vi "Get Completed Log Files.vi"(8 "error in (no error)":errorcluster, 10 "Session Name in":string, 11 "Data Logging Manager Ref in":T1) -> (0 "error out":errorcluster, 1 "Log File Paths":path[](array[path]), 2 "Session Name out":string, 3 "Data Logging Manager Ref out":T1)   [LabVIEW 2020, in "NI_VS Data Logging API.lvlib"]
doc: "Gets the paths to all the log files created during the logging session specified by <B>Session Name in</B>."
uses:
  <vilib>/NI VeriStand/Execution/DataLogging/NI_VS Data Logging API.lvlib
  <vilib>/NI VeriStand/Execution/DataLogging/IDataLogging Ref.ctl
  NationalInstruments.VeriStand.ClientAPI
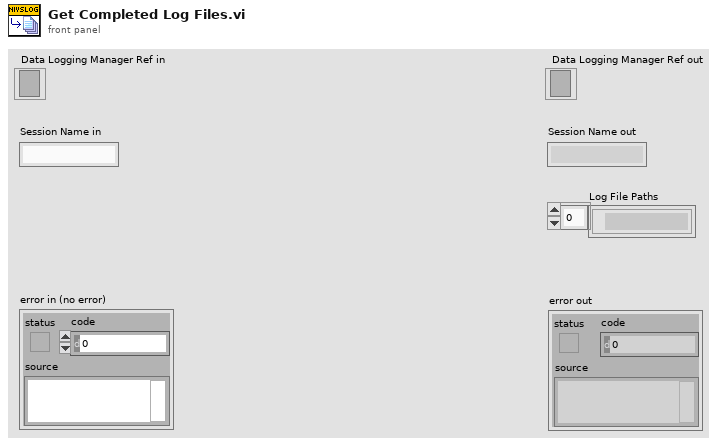
[diagram p1: front panel]
types:
  T1 = typedef "NI_VS Data Logging API.lvlib/IDataLogging Ref.ctl" = refnum<k24>
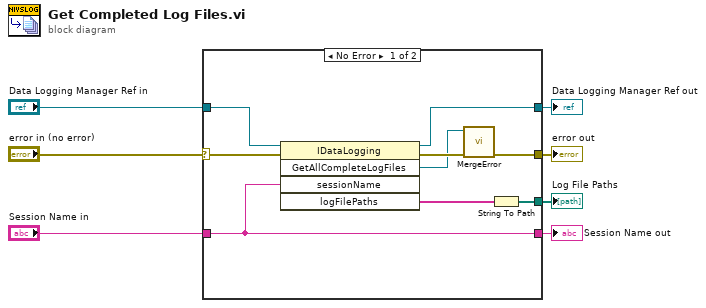
[diagram p0: block diagram]
diagram:
  n1 = case shown="No Error" "error in (no error)" {
    selector: "error in (no error)" -> [w14 w19]
    tunnel: [w11 w19] -> w6
    tunnel: [w10 w18] -> w5
    tunnel: "Data Logging Manager Ref in" -> [w16 w18]
    tunnel: [w15 w17] -> w3
    tunnel: "Session Name in" -> [w15 w17]
    tunnel: [w8 _] -> w1
    frame No Error {
      n2 = invoke class="IDataLogging" method="GetAllCompleteLogFiles"(reference=w16, error in=w14, "sessionName"=w15) -> (reference out=w10:T1, error out=w13:errorcluster, "GetAllCompleteLogFiles"=w12:refnum<k24>, "logFilePaths"=w9:string[])  [unwired: 2 in, 1 out]
      n3 = call <vilib>:"MergeError.vi"("error in (no error)"=w13, "Error"=w12) -> ("error out"=w11:errorcluster)  [unwired: 9 out]
      n4 = String To Path(string=w9) -> (path=w8:path[])
    }
    frame Error {
    }
  }
  "Data Logging Manager Ref out" <- w5
  "error out" <- w6
  "Session Name out" <- w3
  "Log File Paths" <- w1
